vi "Actor Core.vi"(8 "error in":errorcluster caption="错误输入", 11 "客户端 in":refnum<class "客户端.lvclass"> caption="操作者输入") -> (0 "error out":errorcluster caption="错误输出", 3 "Actor out":refnum<class "Actor.lvclass"> caption="操作者输出")   [LabVIEW 2015, in "客户端.lvlib" / "客户端.lvclass"]
doc: "(<B>文件名</B>: Actor Framework.lvlib:Actor.lvclass:Actor Core.vi)\n\n接收发送至操作者的消息，响应消息并处理可能导致操作者关闭的错误。\n\n子孙类重写该VI，使操作者完成特定的任务。使用调用父方法节点实现重写。"
uses:
  <vilib>/ActorFramework/Actor/Actor.lvclass
panel:
  out "硬件返回的数据":string
  out "客户端名称":string
  in  "指令":string
  in  "发送指令":bool
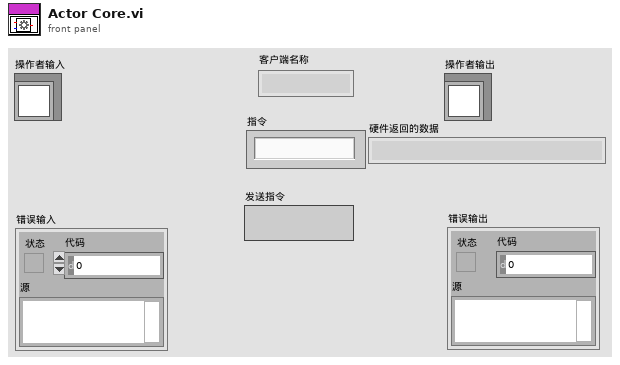
[diagram p1: front panel]
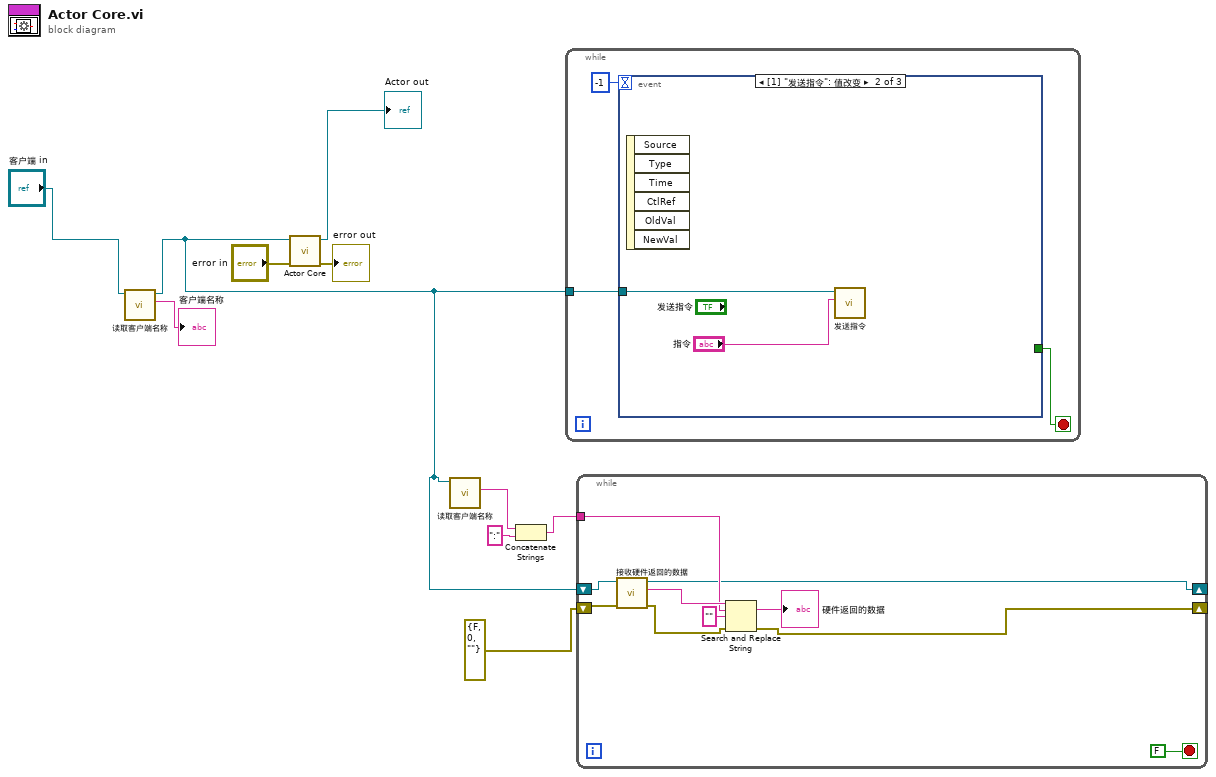
[diagram p0: block diagram]
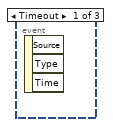
[diagram p2: hidden frame]
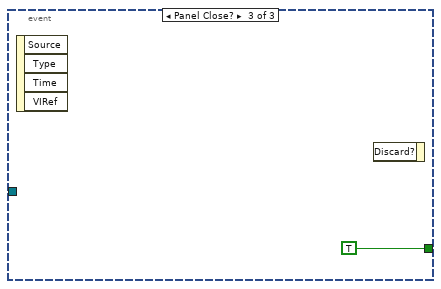
[diagram p3: hidden frame]
diagram:
  n1 = call-dynamic "读取客户端名称.vi"("客户端输入"="客户端 in") -> ("客户端名称"=→"客户端名称":string, "客户端输出"=w2:refnum<class "客户端.lvclass">)  [unwired: 8 in, 1 out]
  n2 = call-parent "Actor Core.vi"("error in"="error in", "Actor in"=w2) -> ("error out"=→"error out":errorcluster, "Actor out"=→"Actor out":refnum<class "Actor.lvclass">)  [unwired: 8 in]
  n3 = call-dynamic "读取客户端名称.vi"("客户端输入"=w2) -> ("客户端名称"=w5:string)  [unwired: 8 in, 2 out]
  n4 = Concatenate Strings(w5, ":" ("字符串")) -> (w3:string)
  n5 = while {
    tunnel: w2 -> [w11]
    stop <- w13 stop-if-true
    n6 = event shown="[1] \"发送指令\": 值改变" {
      selector: _ -> [_ _ _]
      dyn-events: _ -> [_ _ _]
      timeout: -1 -> [_ _ _]
      tunnel: [_ _ TRUE] -> w13
      tunnel: w11 -> [_ w14 _]
      event Timeout {
        n7 = event-data() -> ()  [unwired: 1 in, 3 out]
      }
      event "发送指令": Value Change {
        n8 = event-data() -> ()  [unwired: 1 in, 6 out]
        n9 = call-dynamic "发送指令.vi"("指令"="指令", "客户端 输入"=w14) -> ()  [unwired: 8 in, 2 out]
      }
      event Panel Close? {
        n10 = event-data() -> ()  [unwired: 1 in, 4 out]
        n11 = event-data() -> ()  [unwired: 2 in, 1 out]
      }
    }
  }
  n12 = while {
    tunnel: w3 -> [w23]
    shift-right: [w19] -> _
    shift-left: w2 -> [w20]
    shift-right: [w17] -> _
    shift-left: errorcluster {"status"=FALSE, "code"=0, "source"=""} ("error in") -> [w18]
    stop <- FALSE stop-if-true
    n13 = call-dynamic "接收硬件返回的数据.vi"("error in (no error)"=w18, "客户端 输入"=w20) -> ("error out"=w21:errorcluster, "硬件返回的数据"=w25:string, "客户端 输出"=w19:refnum<class "客户端.lvclass">)  [unwired: 7 in]
    n14 = Search and Replace String(input string=w25, search string=w23, replace string="" ("替换字符串(\"\")"), error in=w21) -> (result string=→"硬件返回的数据":string, error out=w17:errorcluster)  [unwired: 4 in, 2 out]
  }
